vi "2D Eval Func at Sampling Pnts.vi"(6 "VI ref":cluster{"f(X)":refnum<vi>, "data":variant}, 7 "Formula":T1, 8 "error in (no error)":errorcluster, 9 "Formula/VI ref":bool, 10 "y limit":cluster{"y lower":dbl, "y upper":dbl}={"y lower"=0.0, "y upper"=1.0}, 11 "x limit":cluster{"x lower":dbl, "x upper":dbl}={"x lower"=0.0, "x upper"=1.0}) -> (0 "error out":errorcluster, 1 "Sampling points (7-order)":dbl[][](array[numeric]), 2 "Function Evaluations (4 pts)":dbl[][](array[numeric]), 3 "Function Evaluations (7 pts)":dbl[][](array[numeric]))   [LabVIEW 2014, in "NI_AALPro.lvlib"]
uses:
  NI_AALPro.lvlib
  NI_Gmath.lvlib
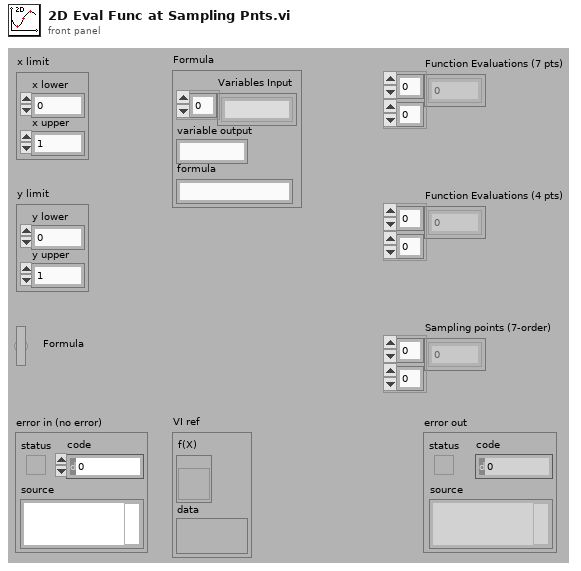
[diagram p1: front panel]
types:
  T1 = cluster{"Variables Input":string[], "variable output":string, "formula":string}
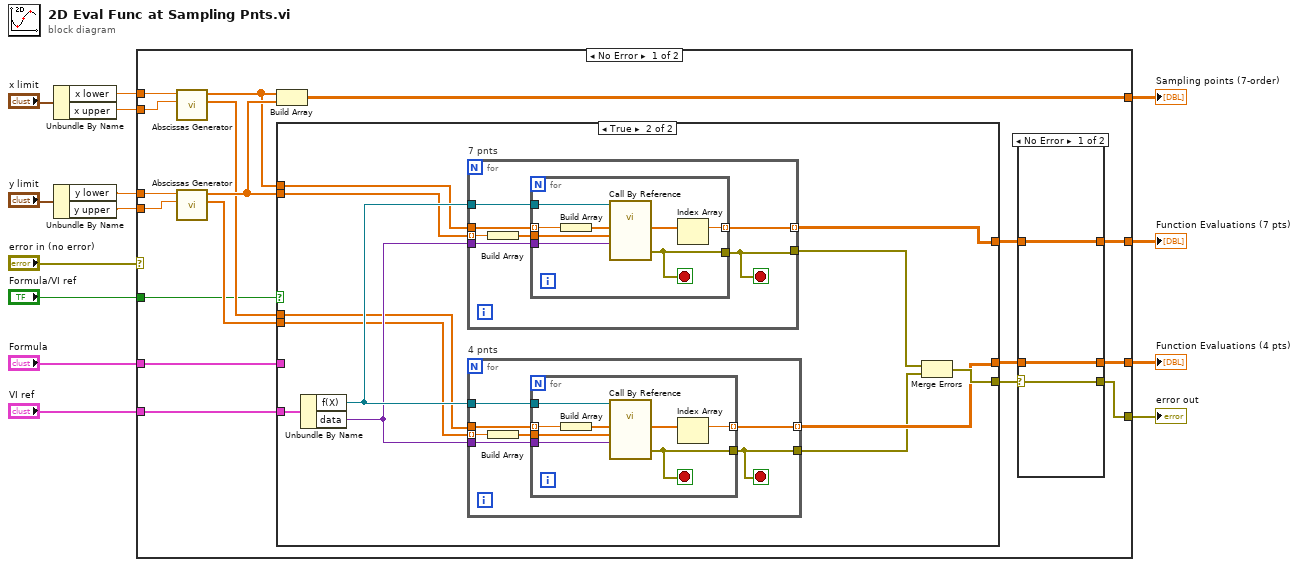
[diagram p0: block diagram]
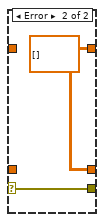
[diagram p2: hidden frame]
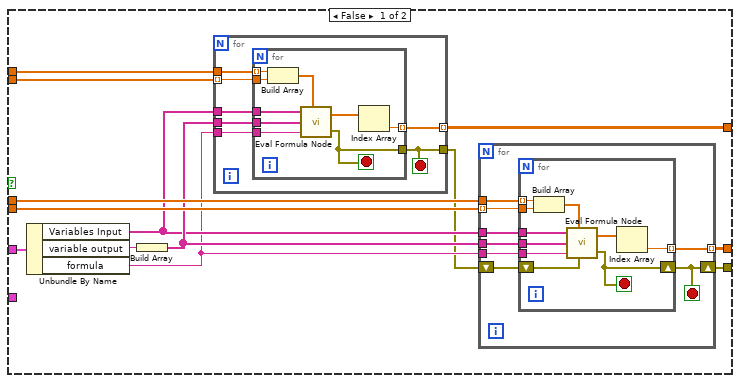
[diagram p3: hidden frame]
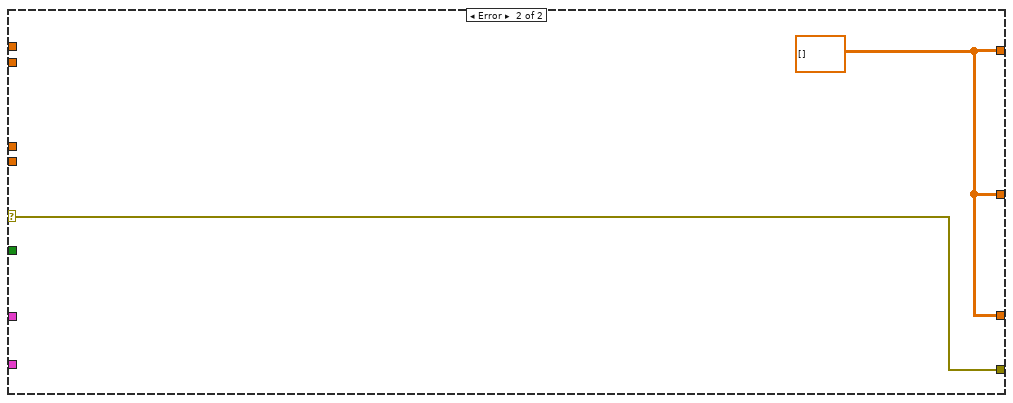
[diagram p4: hidden frame]
diagram:
  n1 = Unbundle By Name("x limit") -> ("x lower"=w9:dbl, "x upper"=w8:dbl)
  n2 = Unbundle By Name("y limit") -> ("y lower"=w6:dbl, "y upper"=w5:dbl)
  n3 = case shown="No Error" "error in (no error)" {
    selector: "error in (no error)" -> [_ w128]
    tunnel: [w26 w127] -> w14
    tunnel: [w15 w127] -> w13
    tunnel: [w19 w128] -> w12
    tunnel: w9 -> [w32 _]
    tunnel: w8 -> [w31 _]
    tunnel: w6 -> [w30 _]
    tunnel: w5 -> [w29 _]
    tunnel: [w16 w127] -> w4
    tunnel: "Formula/VI ref" -> [w23 _]
    tunnel: "Formula" -> [w22 _]
    tunnel: "VI ref" -> [w21 _]
    frame No Error {
      n4 = call "Abscissas Generator.vi"("upper limit"=w31, "lower limit"=w32) -> ("4 points"=w25:dbl[], "7 points"=w27:dbl[])  [unwired: 8 out]
      n5 = call "Abscissas Generator.vi"("upper limit"=w29, "lower limit"=w30) -> ("4 points"=w24:dbl[], "7 points"=w28:dbl[])  [unwired: 8 out]
      n6 = Build Array(w27, w28) -> (w26:dbl[][])
      n7 = case shown="True" w23 {
        tunnel: [w50 w94] -> w17
        tunnel: w28 -> [w49 w92]
        tunnel: w27 -> [w48 w91]
        tunnel: w25 -> [w47 w88]
        tunnel: w24 -> [w46 w87]
        tunnel: [w45 w93] -> w18
        tunnel: [w43 w95] -> w20
        tunnel: w22 -> [w42 _]
        tunnel: w21 -> [_ w90]
        frame False {
          n8 = Unbundle By Name(w42) -> ("Variables Input"=w40:string[], "variable output"=w41:string, "formula"=w39:string)
          n9 = Build Array(w41) -> (w44:string[])
          n10 = for {
            tunnel: [w57] -> w50 mode=indexing
            tunnel: w49 -> [w56] mode=indexing
            tunnel: w48 -> [w55]
            tunnel: w40 -> [w54]
            tunnel: w44 -> [w53]
            tunnel: w39 -> [w52]
            tunnel: [w51] -> w38
            stop <- w51 stop-if-true
            n11 = for {
              tunnel: w52 -> [w66]
              tunnel: w54 -> [w65]
              tunnel: w53 -> [w64]
              tunnel: w55 -> [w63] mode=indexing
              tunnel: [w62] -> w57 mode=indexing
              tunnel: w56 -> [w59]
              tunnel: [w58] -> w51
              stop <- w58 stop-if-true
              n12 = Build Array(w63, w59) -> (w60:dbl[])
              n13 = call "Eval Formula Node.vi"("Variables Input"=w65, "Input Values"=w60, "Variables Output"=w64, "formula"=w66) -> ("Output Values"=w61:dbl[], "error out"=w58:errorcluster)  [unwired: 1 in]
              n14 = Index Array(array=w61) -> (element=w62:dbl)  [unwired: 1 in]
            }
          }
          n15 = for {
            tunnel: w47 -> [w74]
            tunnel: w46 -> [w73] mode=indexing
            tunnel: w40 -> [w72]
            tunnel: w44 -> [w71]
            tunnel: w39 -> [w70]
            tunnel: [w69] -> w45 mode=indexing
            shift-right: [w67] -> w43
            shift-left: w38 -> [w68]
            stop <- w67 stop-if-true
            n16 = for {
              tunnel: w70 -> [w84]
              tunnel: w72 -> [w83]
              tunnel: w71 -> [w82]
              tunnel: w74 -> [w81] mode=indexing
              tunnel: [w80] -> w69 mode=indexing
              tunnel: w73 -> [w76]
              shift-right: [w75] -> w67
              shift-left: w68 -> [w78]
              stop <- w75 stop-if-true
              n17 = Build Array(w81, w76) -> (w77:dbl[])
              n18 = call "Eval Formula Node.vi"("Variables Input"=w83, "Input Values"=w77, "Variables Output"=w82, "formula"=w84, "error in (no error)"=w78) -> ("Output Values"=w79:dbl[], "error out"=w75:errorcluster)
              n19 = Index Array(array=w79) -> (element=w80:dbl)  [unwired: 1 in]
            }
          }
        }
        frame True {
          n20 = Unbundle By Name(w90) -> ("f(X)"=w96:refnum<vi>, "data"=w89:variant)
          n21 = for "7 pnts" {
            tunnel: w96 -> [w118]
            tunnel: [w112] -> w86
            tunnel: w89 -> [w117]
            tunnel: [w116] -> w94 mode=indexing
            tunnel: w91 -> [w115]
            tunnel: w92 -> [w114] mode=indexing
            stop <- w112 stop-if-true
            n22 = Build Array(w114) -> (w113:dbl[])
            n23 = for {
              tunnel: w118 -> [w126]
              tunnel: [w119] -> w112
              tunnel: w117 -> [w125]
              tunnel: [w120] -> w116 mode=indexing
              tunnel: w115 -> [w123] mode=indexing
              tunnel: w113 -> [w122]
              stop <- w119 stop-if-true
              n24 = Build Array(w123) -> (w121:dbl[])
              n25 = call-by-ref "?"(reference=w126, "data"=w125, "Y"=w122, "X"=w121) -> ("error out"=w119:errorcluster, "F(X,Y)"=w124:dbl[])  [unwired: 8 in, 2 out]
              n26 = Index Array(array=w124) -> (element=w120:dbl)  [unwired: 1 in]
            }
          }
          n27 = for "4 pnts" {
            tunnel: w96 -> [w103]
            tunnel: [w97] -> w85
            tunnel: w89 -> [w102]
            tunnel: [w101] -> w93 mode=indexing
            tunnel: w88 -> [w100]
            tunnel: w87 -> [w99] mode=indexing
            stop <- w97 stop-if-true
            n28 = Build Array(w99) -> (w98:dbl[])
            n29 = for {
              tunnel: w103 -> [w111]
              tunnel: w102 -> [w110]
              tunnel: [w105] -> w101 mode=indexing
              tunnel: w100 -> [w108] mode=indexing
              tunnel: w98 -> [w107]
              tunnel: [w104] -> w97
              stop <- w104 stop-if-true
              n30 = Build Array(w108) -> (w106:dbl[])
              n31 = call-by-ref "?"(reference=w111, "data"=w110, "Y"=w107, "X"=w106) -> ("error out"=w104:errorcluster, "F(X,Y)"=w109:dbl[])  [unwired: 8 in, 2 out]
              n32 = Index Array(array=w109) -> (element=w105:dbl)  [unwired: 1 in]
            }
          }
          n33 = Merge Errors(w86, w85) -> (w95:errorcluster)
        }
      }
      n34 = case shown="No Error" w20 {
        selector: w20 -> [w35 w37]
        tunnel: [w35 w37] -> w19
        tunnel: w18 -> [w34 _]
        tunnel: w17 -> [w33 _]
        tunnel: [w34 w36] -> w16
        tunnel: [w33 w36] -> w15
        frame No Error {
        }
        frame Error {
          w36 = dbl[][] []
        }
      }
    }
    frame Error {
      w127 = dbl[][] []
    }
  }
  "Sampling points (7-order)" <- w14
  "Function Evaluations (7 pts)" <- w13
  "error out" <- w12
  "Function Evaluations (4 pts)" <- w4
